vi "Data log test.vi"() -> ()   [LabVIEW 2017]
uses:
  <vilib>/rvi/interface/nirviOpenFPGA/nirviOpenFPGA.xnode
  <vilib>/rvi/interface/nirviMethod/nirviMethod.xnode
  <vilib>/rvi/interface/nirviReadWriteControl/nirviReadWriteControl.xnode
  <vilib>/FPGAPlugInAG/Dynamic/niLvFpga_Run_Dynamic.vi
  <vilib>/FPGAPlugInAG/Dynamic/niLvFpga_Reset_Dynamic.vi
  <vilib>/FPGAPlugInAG/Dynamic/niLvFpga_ReadFifo_Dynamic.vi
  <vilib>/rvi/errors/niLvFpgaMergeErrorWithErrorCode.vi
  FPGA Bitfiles/Mainproject_FPGATarget_Icreadout_TtJ0N5ODyx0.lvbitx
  Ic readout.vi
  <vilib>/FPGAPlugInAG/cRIO-9063/niLvFpga_Open_cRIO-9063.vi
  <vilib>/rvi/interface/common/dynamic/niFpgaDynamicAddResources.vi
  NiFpgaLv.dll
  <vilib>/Utility/error.llb/Error Cluster From Error Code.vi
  <vilib>/rvi/interface/Simulation/niFpgaSimulationCallBeginRW.vi
  <vilib>/rvi/errors/niLvFpgaAdjustHostInterfaceError.vi
panel:
  in  "Record Samples":u32
  in  "Record PreTrigger Samples":u32
  out "Elements Remaining":u32
  in  "AI Trigger Configuration":T1
  in  "Points get":i32=100
  out "Data":fxp<+/-,17,5>[](array[numeric])=[0.5, 0.5, 0.5, 0.5, 0.5, 0.5, 0.5, 0.5, 0.5, 0.5]
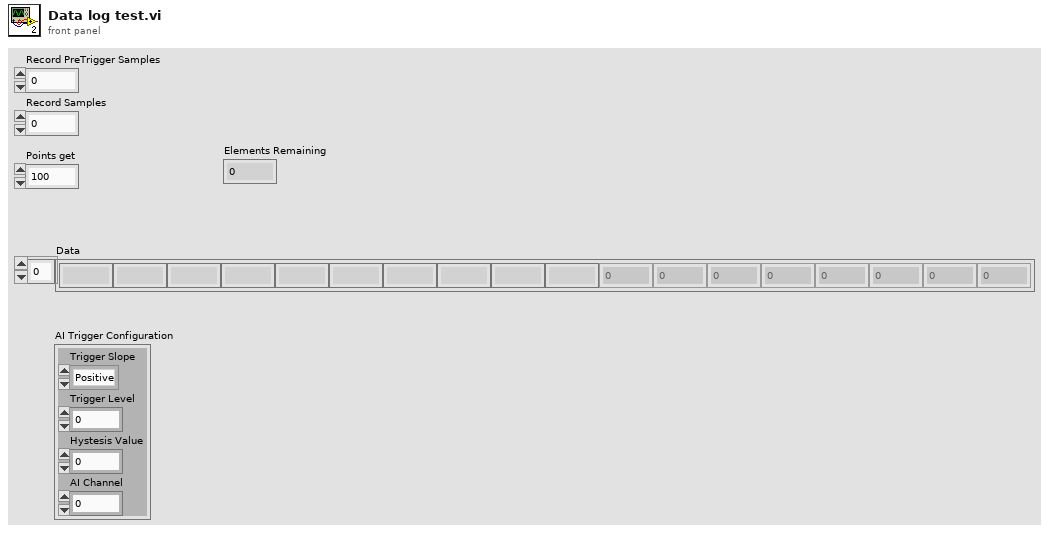
[diagram p1: front panel]
types:
  T1 = cluster{"Trigger Slope":enum8{"Positive", "Negative"}, "Trigger Level":fxp<+/-,17,5>, "Hystesis Value":fxp<+,16,4>, "AI Channel":u8}
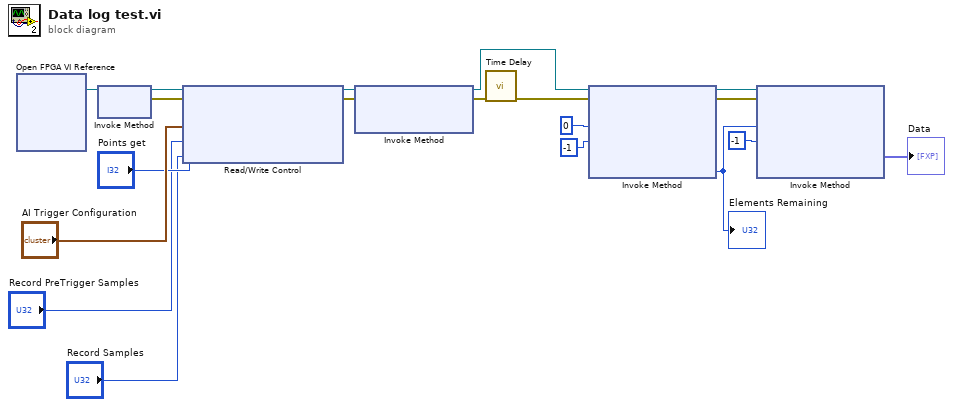
[diagram p0: block diagram]
diagram:
  n1 = xnode "Open FPGA VI Reference"() -> ("FPGA VI Reference Out"=w15:refnum<k20>)  [unwired: 2 in, 1 out]
  n2 = xnode "Invoke Method"("FPGA VI Reference In"=w15) -> ("FPGA VI Reference Out"=w14:refnum<k20>, "error out"=w13:errorcluster)  [unwired: 1 in]
  n3 = xnode "Read/Write Control"("FPGA VI Reference In"=w14, "error in"=w13, "Points"="Points get", "AI Trigger Configuration"="AI Trigger Configuration", "Record PreTrigger Samples"="Record PreTrigger Samples", "Record Samples"="Record Samples") -> ("FPGA VI Reference Out"=w18:refnum<k20>, "error out"=w3:errorcluster)
  n4 = xnode "Invoke Method"("FPGA VI Reference In"=w18, "error in"=w3) -> ("FPGA VI Reference Out"=w11:refnum<k20>, "error out"=w9:errorcluster)  [unwired: 1 in]
  n5 = call "Time Delay"("error in (no error)"=w9) -> ("error out"=w4:errorcluster)  [unwired: 10 in]
  n6 = xnode "Invoke Method"("FPGA VI Reference In"=w11, "error in"=w4, "Number of Elements"=u32 0, "Timeout (ms)"=-1) -> ("FPGA VI Reference Out"=w10:refnum<k20>, "error out"=w8:errorcluster, "Elements Remaining"=w6:u32)  [unwired: 1 out]
  "Elements Remaining" <- w6
  n7 = xnode "Invoke Method"("FPGA VI Reference In"=w10, "error in"=w8, "Number of Elements"=w6, "Timeout (ms)"=-1) -> ("Data"=→"Data":fxp<+/-,17,5>[])  [unwired: 3 out]
